vi "GT Print Watch.vi"(7 "printCount":u32, 8 "error in (no error)":errorcluster caption="错误输入（无错误）", 9 "start":i32, 10 "pFileName":string, 11 "cardNum":i16) -> (0 "error out":errorcluster caption="错误输出", 3 "function return":i16)   [LabVIEW 2020, in "gts1.lvlib"]
doc: "GT_API GT_PrintWatch(short cardNum,const char *pFileName,long start=0,unsigned long printCount=0);"
uses:
  gts1.lvlib
  dll/32bit/multi_card/gts.dll
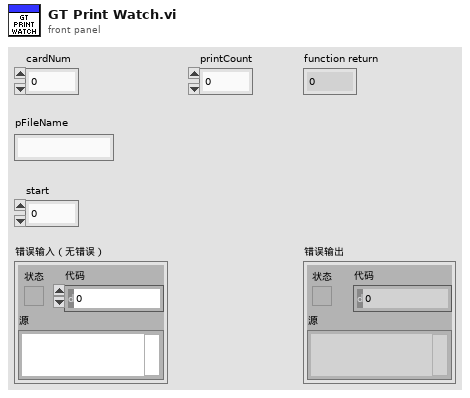
[diagram p1: front panel]
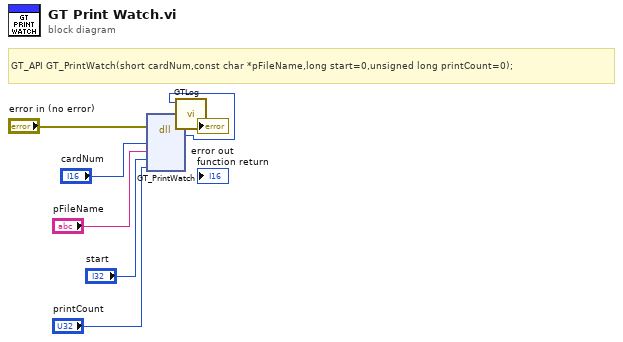
[diagram p0: block diagram]
diagram:
  # "GT_API GT_PrintWatch(short cardNum,const char *pFileName,long start=0,unsigned long printCount=0);"
  n1 = dll-call lib="C:/1228/dll/32bit/multi_card/gts.dll" fn="GT_PrintWatch"(error in="error in (no error)", "cardNum"="cardNum", "pFileName"="pFileName", "start"="start", "printCount"="printCount") -> (error out=w3:errorcluster, w1:i16)  [unwired: 6 in, 1 out]
  n2 = call "GTLog.vi"("error in (no error)"=w3, "Numeric"=w1) -> ("error out"=→"error out":errorcluster)  [unwired: 9 in]
